vi "Flatten.vi"(8 "error in":errorcluster, 9 "Data":T1) -> (0 "error out":errorcluster, 2 "Buffer":u8[](array[numeric]) format="%.0x")   [LabVIEW 2020, in "TcpServerHello.lvlib"]
uses:
  TcpServerHello.lvlib
  Data.ctl
  ConnectStatus/ConnectStatus.lvlib
  ConnectStatus/Enumeration.ctl
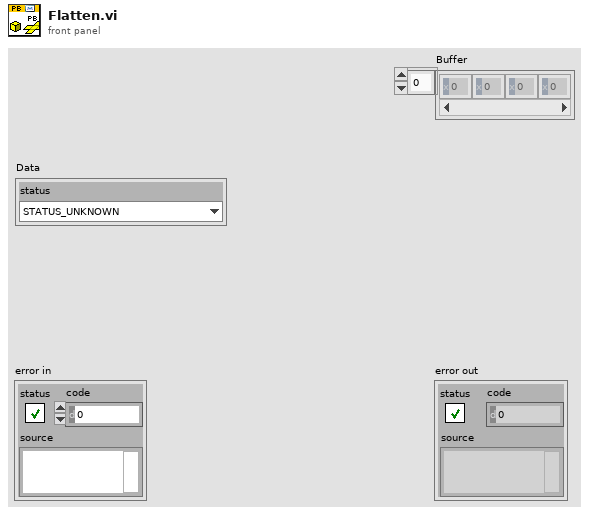
[diagram p1: front panel]
types:
  T1 = typedef "TcpServerHello.lvlib/Data.ctl" = cluster{"status":T2}
  T2 = typedef "ConnectStatus.lvlib/Enumeration.ctl" = enum16{"STATUS_UNKNOWN", "STATUS_SUCCESS", "STATUS_ERROR", "STATUS_BAD_CONFIG", "STATUS_BAD_SYSTEM", "STATUS_BAD_CLUSTER"}
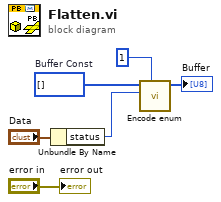
[diagram p0: block diagram]
diagram:
  w4 = u8[] []  # Buffer Const
  n1 = Unbundle By Name("Data") -> ("status"=w2:T2)
  n2 = call "Encode enum.vi"("Field Number"=1, "Enumeration"=w2, "Buffer in"=w4) -> ("Buffer"=→"Buffer":u8[])  [unwired: 8 in]
  "error out" <- "error in"
